vi "generate timelapse table.vi"(8 "error in (no error)":errorcluster, 11 "Tomo in":refnum<class "Tomo.lvclass">) -> (0 "error out":errorcluster, 2 "timelapse table":dbl[][](array[numeric]), 3 "Tomo out":refnum<class "Tomo.lvclass">)   [LabVIEW 2012, in "Tomo.lvclass"]
uses:
  Tomo.lvclass
  Tomo.lvclass/Tomo.ctl
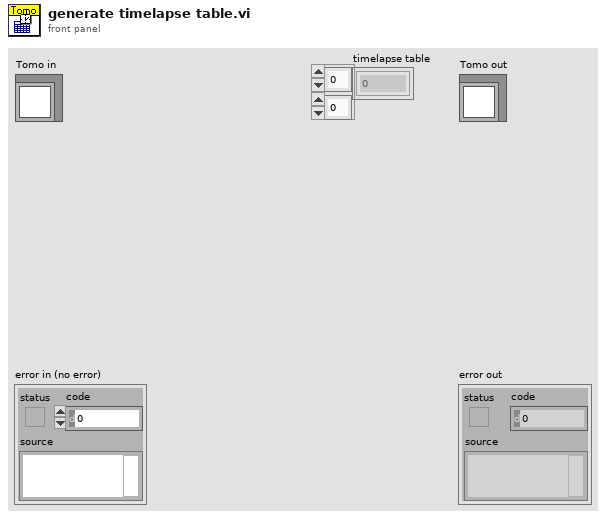
[diagram p1: front panel]
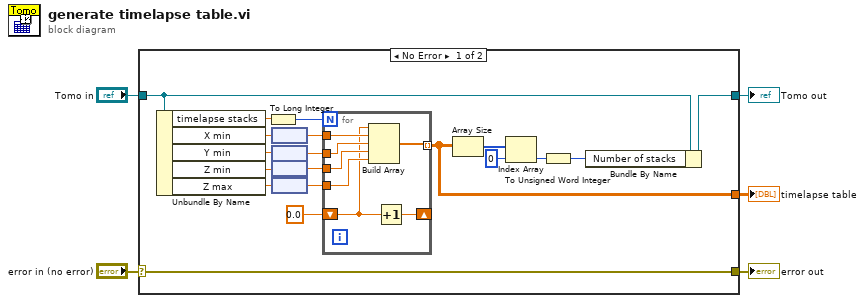
[diagram p0: block diagram]
diagram:
  n1 = case shown="No Error" "error in (no error)" {
    selector: "error in (no error)" -> [w24 w33]
    tunnel: [w24 w33] -> w4
    tunnel: [w9 w32] -> w2
    tunnel: "Tomo in" -> [w10 w32]
    tunnel: [w6 _] -> w1
    frame No Error {
      n2 = Unbundle By Name(w10) -> ("timelapse stacks"=w23:dbl, "X min"=w21:dbl[unit], "Y min"=w19:dbl[unit], "Z min"=w18:dbl[unit], "Z max"=w17:dbl[unit])
      n3 = To Long Integer(number=w23) -> (32bit integer=w22:i32)
      n4 = node(w21) -> (w20:dbl)
      n5 = node(w19) -> (w16:dbl)
      n6 = node(w18) -> (w15:dbl)
      n7 = node(w17) -> (w14:dbl)
      n8 = for {
        N: w22 -> [_]
        tunnel: w20 -> [w31]
        tunnel: w16 -> [w30]
        tunnel: w15 -> [w29]
        tunnel: w14 -> [w28]
        shift-right: [w27] -> _
        shift-left: 0.0 -> [w26]
        tunnel: [w25] -> w6 mode=indexing
        n9 = Build Array(w26, w31, w30, w29, w28) -> (w25:dbl[])
        n10 = Increment(x=w26) -> (x+1=w27:dbl)
      }
      n11 = Array Size(array=w6) -> (size(s)=w12:i32[])
      n12 = Index Array(array=w12, index=0) -> (element=w8:i32)
      n13 = To Unsigned Word Integer(number=w8) -> (unsigned 16bit integer=w7:u16)
      n14 = Bundle By Name(cluster=w10, "Number of stacks"=w7) -> (w9:refnum<class "Tomo.lvclass">)
    }
    frame Error {
    }
  }
  "error out" <- w4
  "Tomo out" <- w2
  "timelapse table" <- w1
